vi "Win32-Window Always On Top.vi"(8 "error in (no error)":errorcluster, 11 "VI reference":refnum<vi>) -> (0 "error out":errorcluster, 3 "VI ref out":refnum<vi>)   [LabVIEW 2020]
doc: "Uses Windows API to force panel to stay on top of all other windows."
uses:
  user32.dll
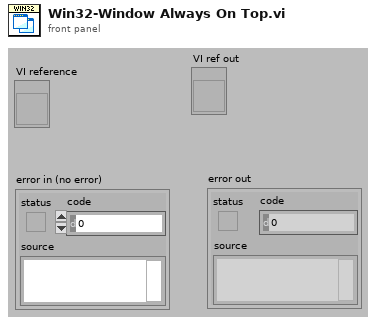
[diagram p1: front panel]
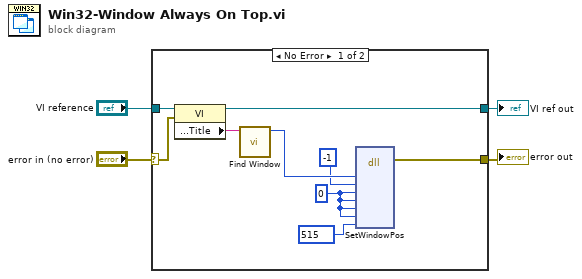
[diagram p0: block diagram]
diagram:
  n1 = case shown="No Error" "error in (no error)" {
    selector: "error in (no error)" -> [w6 w15]
    tunnel: "VI reference" -> [w8 w14]
    tunnel: [w7 w15] -> w3
    tunnel: [w5 w14] -> w1
    frame No Error {
      w11 = 0 ("X")
      n2 = property class="VI"(reference=w8, error in=w6) -> (reference out=w5:refnum<vi>, "Front Panel.Title"=w13:string)  [unwired: 1 out]
      n3 = call "Find Window.vi"("Window Name"=w13) -> ("Win32 Window Handle"=w12:i32)  [unwired: 9 in, 1 out]
      n4 = dll-call lib="user32.dll" fn="SetWindowPos"("hWnd"=w12, "hWndInsertAfter"=-1, "X"=w11, "Y"=w11, "cx"=w11, "cy"=w11, "uFlags"=u32 515) -> (error out=w7:errorcluster)  [unwired: 10 in, 2 out]
    }
    frame Error {
    }
  }
  "error out" <- w3
  "VI ref out" <- w1
